vi "Expansion of hills.vi"(1 "Q Radius":i16, 2 "SICK Threshold":i16, 3 "Actual SICK":i16[](array[numeric])) -> (0 "Modified Binary SICK":i16[](array[numeric]))   [LabVIEW 2009]
doc: "This VI takes raw SICK data and creates a binary histogram with expanded hills."
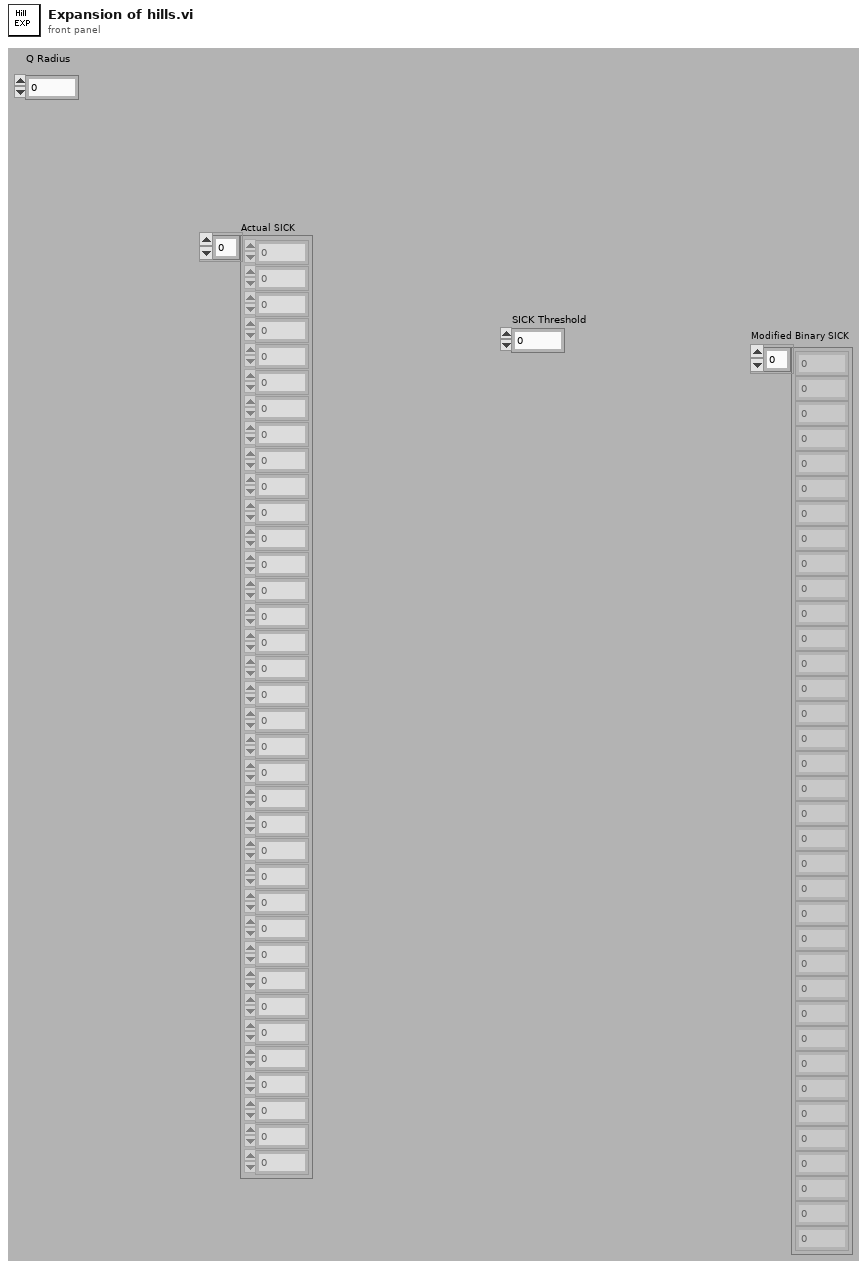
[diagram p1: front panel]
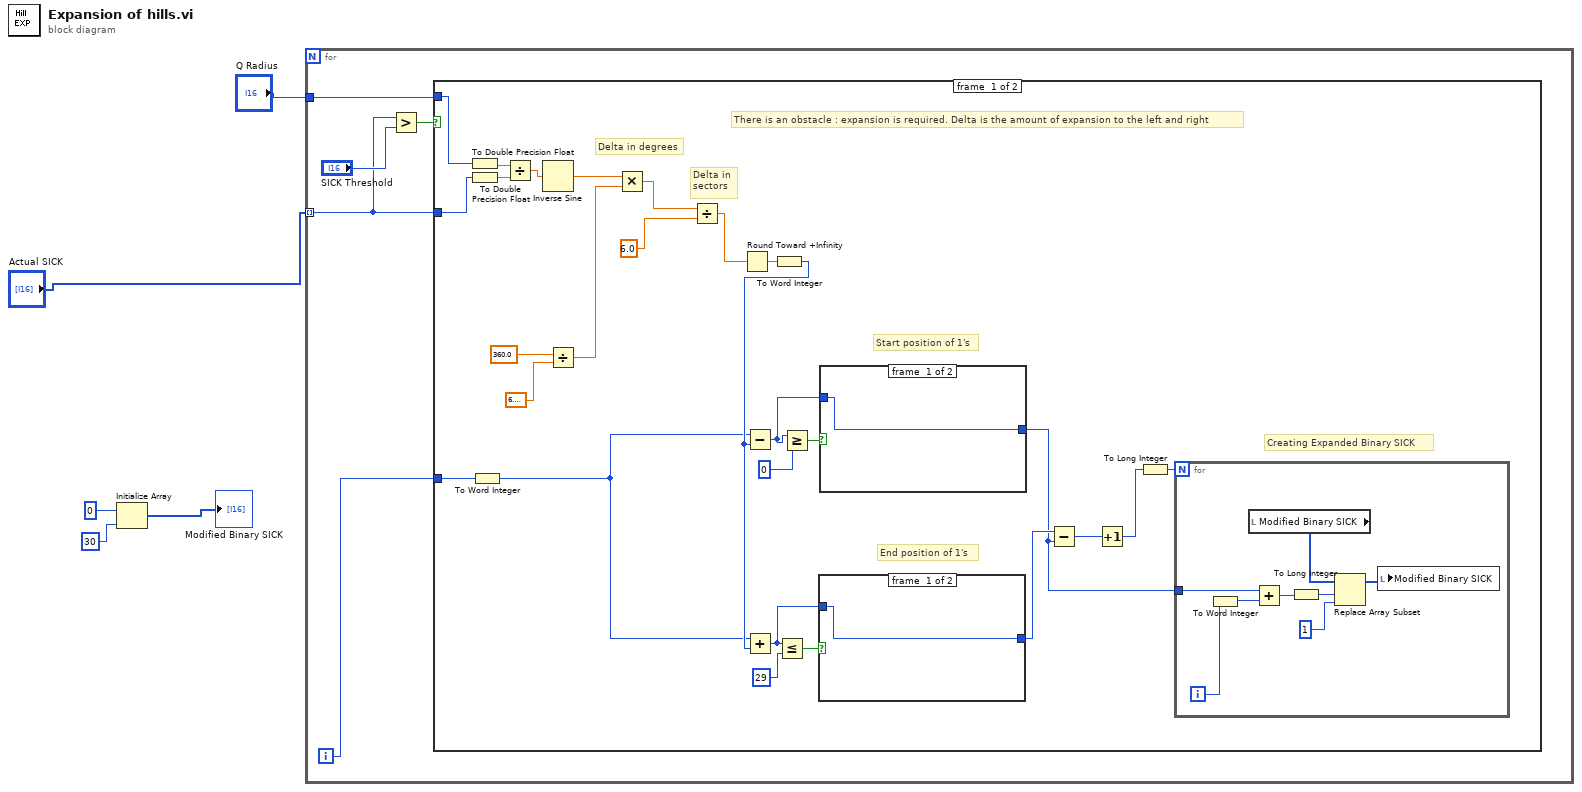
[diagram p0: block diagram]
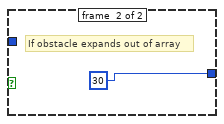
[diagram p2: hidden frame]
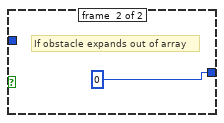
[diagram p3: hidden frame]
diagram:
  n1 = Initialize Array(i16 0 ("element"), 30 ("dimension size")) -> (→"Modified Binary SICK":i16[])
  n2 = for {
    tunnel: "Actual SICK" -> [w6] mode=indexing
    tunnel: "Q Radius" -> [w10]
    i -> [w7]
    n3 = Greater?(x=w6, y="SICK Threshold") -> (0:w8:bool)
    n4 = case shown="False" w8 {
      tunnel: w10 -> [w19 _]
      tunnel: w7 -> [w14 _]
      tunnel: w6 -> [w17 _]
      frame #0 {
        # "Creating Expanded Binary SICK"
        # "End position of 1's"
        # "Start position of 1's"
        # "Delta in \nsectors"
        # "Delta in degrees"
        # "There is an obstacle : expansion is required. Delta is the amount of expansion to the left and right"
        n5 = To Double Precision Float(number=w19) -> (double precision float=w20:dbl)
        n6 = To Double Precision Float(number=w17) -> (double precision float=w18:dbl)
        n7 = To Word Integer(number=w14) -> (16bit integer=w13:i16)
        n8 = Divide(x=w20, y=w18) -> (x/y=w37:dbl)
        n9 = Inverse Sine(1:w37) -> (0:w36:dbl)
        n10 = Divide(x=360.0 ("y"), y=6.283185307179586) -> (x/y=w33:dbl)
        n11 = Multiply(x=w36, y=w33) -> (x*y=w32:dbl)
        n12 = Divide(x=w32, y=6.0) -> (x/y=w30:dbl)
        n13 = Round Toward +Infinity(x=w30) -> (ceil(x): smallest int >= x=w16:dbl)
        n14 = To Word Integer(number=w16) -> (16bit integer=w15:i16)
        n15 = Subtract(x=w13, y=w15) -> (x-y=w24:i16)
        n16 = Add(x=w13, y=w15) -> (x+y=w28:i16)
        n17 = Less Or Equal?(x=w28, y=i16 29) -> (x <= y?=w29:bool)
        n18 = Greater Or Equal?(x=w24, y=i16 0) -> (x >= y?=w23:bool)
        n19 = case shown="False" w29 {
          tunnel: [w46 i16 30] -> w27
          tunnel: w28 -> [w46 _]
          frame #0 {
          }
          frame #1 {
            # "If obstacle expands out of array"
          }
        }
        n20 = case shown="False" w23 {
          tunnel: [w48 i16 0] -> w25
          tunnel: w24 -> [w48 _]
          frame #0 {
          }
          frame #1 {
            # "If obstacle expands out of array"
          }
        }
        n21 = Subtract(x=w27, y=w25) -> (x-y=w26:i16)
        n22 = Increment(x=w26) -> (x+1=w11:i16)
        n23 = To Long Integer(number=w11) -> (32bit integer=w12:i32)
        n24 = for {
          N: w12 -> [_]
          tunnel: w25 -> [w42]
          i -> [w40]
          n25 = To Word Integer(number=w40) -> (16bit integer=w41:i16)
          n26 = local read "Modified Binary SICK"() -> (w44:i16[])
          n27 = Add(x=w42, y=w41) -> (x+y=w39:i16)
          n28 = To Long Integer(number=w39) -> (32bit integer=w38:i32)
          n29 = Replace Array Subset(array=w44, new element=i16 1, index=w38) -> (w43:i16[])
          n30 = local write "Modified Binary SICK"(w43) -> ()
        }
      }
      frame #1 {
        # "Open Valley\nNo expansion"
      }
    }
  }
